vi "Default Settings.vi"(8 "error in (no error)":errorcluster, 11 "6 inch CAD Dispense in":refnum<class "6 Inch Sensor Dispense.lvclass">) -> (0 "error out":errorcluster, 3 "6 inch CAD Dispense out":refnum<class "6 Inch Sensor Dispense.lvclass">)   [LabVIEW 2016, in "6 Inch Sensor Dispense.lvclass"]
uses:
  6 Inch Sensor Dispense.lvclass
  C:/Users/HEP Gantry/Documents/GitHub/UCSB-Gantry/V5/Classes/Routine/Dispense/CAD Dispense/Sensor Dispense.lvclass
  C:/Users/HEP Gantry/Documents/GitHub/UCSB-Gantry/V5/Classes/Routine/Dispense/Dispense.lvclass
  Sensor Dispense.lvclass/Sensor Dispense.ctl
  Read Glue Speed.vi
  Read Move Speed.vi
  Sensor Dispense.lvclass
  Dispense.lvclass
panel:
  # "This Routine does not Accept Settings"
  # "This Routine Does not Accept Settings"
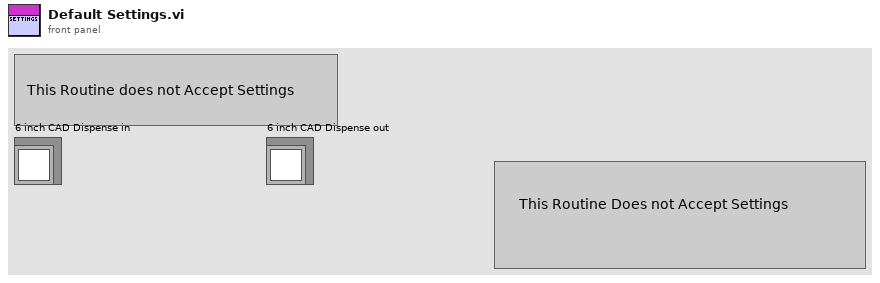
[diagram p1: front panel]
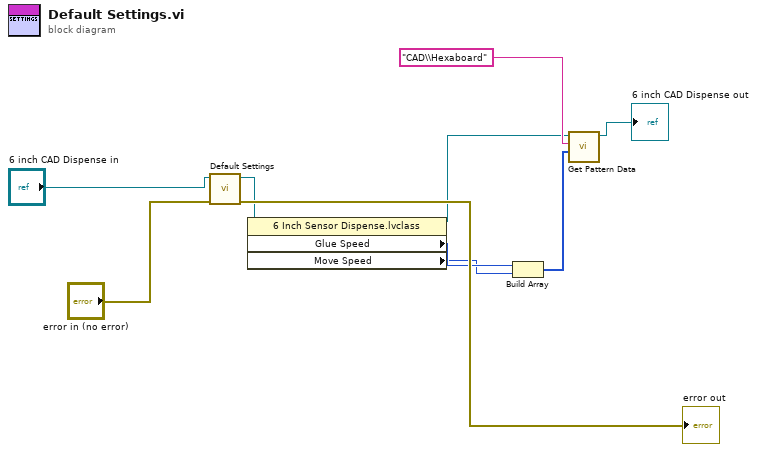
[diagram p0: block diagram]
diagram:
  n1 = call-parent "Default Settings.vi"("error in (no error)"="error in (no error)", "CAD Dispense in"="6 inch CAD Dispense in") -> ("error out"=→"error out":errorcluster, "CAD Dispense out"=w7:refnum<class "6 Inch Sensor Dispense.lvclass">)  [unwired: 8 in]
  n2 = property class="6 Inch Sensor Dispense.lvclass"(reference=w7) -> (reference out=w1:refnum<class "6 Inch Sensor Dispense.lvclass">, "Glue Speed"=w6:i32, "Move Speed"=w5:i32)  [unwired: 1 in, 1 out]
  n3 = Build Array "Build Array"(w6, w5) -> (w4:i32[])
  n4 = call "Get Pattern Data.vi"("File Name"=w4, "Folder Name"="CAD\\Hexaboard", "Dispense.lvclass"=w1) -> ("Dispense Out"=→"6 inch CAD Dispense out":refnum<class "6 Inch Sensor Dispense.lvclass">)  [unwired: 8 in]
